vi "Activation Energies for 20201230.vi"() -> ()   [LabVIEW 2020]
uses:
  <vilib>/Analysis/NI_AALPro.lvlib
panel:
  in  "1/Temp 1D":dbl[](array[numeric])
  in  "ln|dG/dt| 1D":dbl[](array[numeric]) caption="ln|dG/dt|"
  out "E_a 1D HT":dbl
  in  "1/Temp lower temps 1D":dbl[](array[numeric])
  in  "ln|dG/dt| lower temps 1D":dbl[](array[numeric])
  out "E_a 1D":dbl
  out "Arrhenius 1D":T1(graph)
  out "Arrhenius":T1(graph)
  out "E_a 2":dbl
  in  "ln|dG/dt| lower temps":dbl[](array[numeric])
  in  "1/Temp lower temps":dbl[](array[numeric])
  out "E_a":dbl
  in  "ln|dG/dt|":dbl[](array[numeric])
  in  "1/Temp":dbl[](array[numeric])
  # "0.002817\t\n0.002778\t\n0.00274\t\n0.002703\t\n0.002667\t\n0.002632"
  # "0.003509\t\n0.003448\t\n0.00339\t\n0.003333\t\n0.003279\t\n0.003226\t\n0.003175\t\n0.003125\t\n0.003077\t\n0.00303"
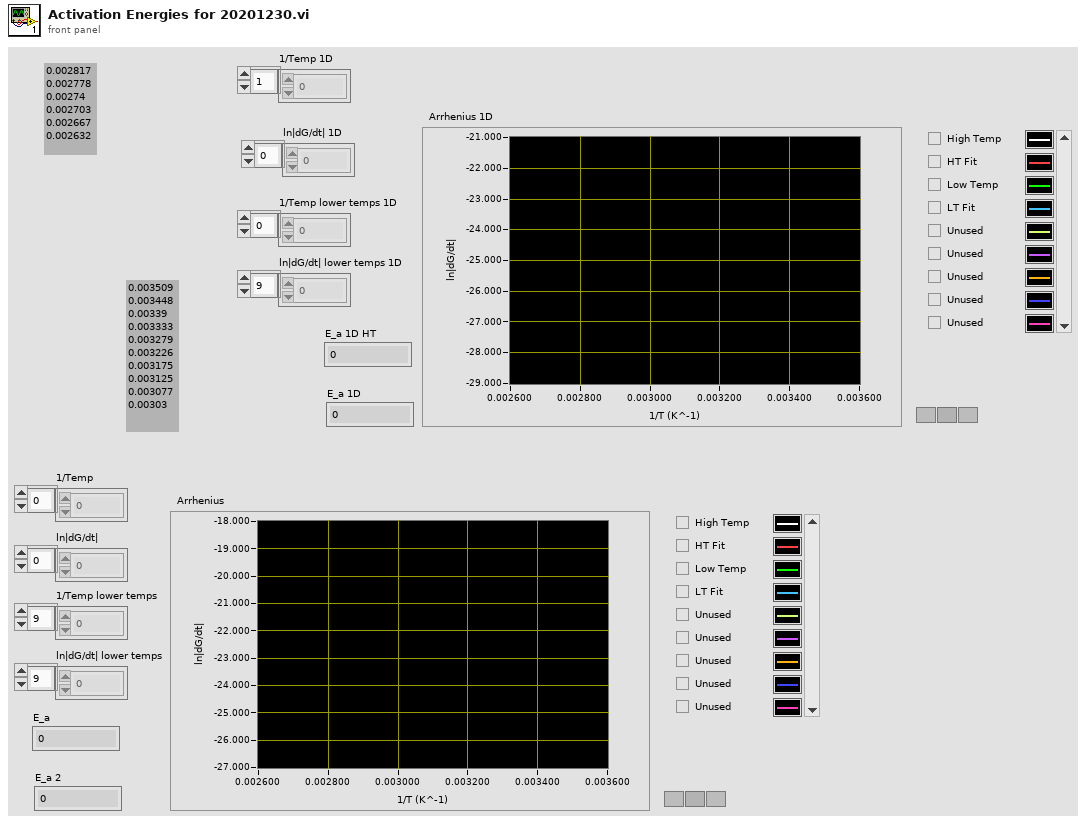
[diagram p1: front panel]
types:
  T1 = cluster{"Data":dbl[], "Best Exponential Fit":dbl[]}[]
  T2 = cluster{"1/Temp 1D":dbl[], "Best Linear Fit":dbl[]}
  T3 = cluster{"1/Temp lower temps 1D":dbl[], "ln|dG/dt| lower temps 1D":dbl[]}
  T4 = cluster{"1/Temp lower temps 1D":dbl[], "Best Linear Fit":dbl[]}
  T5 = cluster{"1/Temp lower temps 1D":dbl[], "Best Linear Fit":dbl[]}[]
  T6 = cluster{"1/Temp lower temps":dbl[], "ln|dG/dt| lower temps":dbl[]}
  T7 = cluster{"1/Temp lower temps":dbl[], "Best Linear Fit":dbl[]}
  T8 = cluster{"1/Temp lower temps":dbl[], "Best Linear Fit":dbl[]}[]
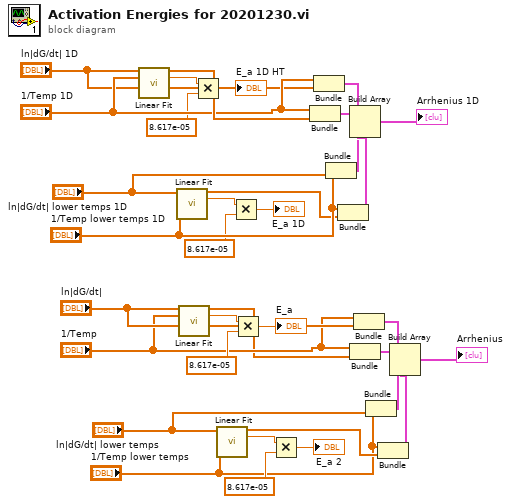
[diagram p0: block diagram]
diagram:
  n1 = call <vilib>:"Linear Fit.vi"("Y"="ln|dG/dt| 1D", "X"="1/Temp 1D") -> ("Best Linear Fit"=w15:dbl[], "slope"=w1:dbl)  [unwired: 9 in, 3 out]
  n2 = call <vilib>:"Linear Fit.vi"("Y"="ln|dG/dt| lower temps 1D", "X"="1/Temp lower temps 1D") -> ("Best Linear Fit"=w12:dbl[], "slope"=w6:dbl)  [unwired: 9 in, 3 out]
  n3 = call <vilib>:"Linear Fit.vi"("Y"="ln|dG/dt|", "X"="1/Temp") -> ("Best Linear Fit"=w20:dbl[], "slope"=w34:dbl)  [unwired: 9 in, 3 out]
  n4 = Multiply(x=w1, y=8.617e-05) -> (x*y=→"E_a 1D HT":dbl)
  n5 = call <vilib>:"Linear Fit.vi"("Y"="ln|dG/dt| lower temps", "X"="1/Temp lower temps") -> ("Best Linear Fit"=w23:dbl[], "slope"=w29:dbl)  [unwired: 9 in, 3 out]
  n6 = Multiply(x=w6, y=8.617e-05) -> (x*y=→"E_a 1D":dbl)
  n7 = Multiply(x=w34, y=8.617e-05) -> (x*y=→"E_a":dbl)
  n8 = Multiply(x=w29, y=8.617e-05) -> (x*y=→"E_a 2":dbl)
  n9 = Bundle("1/Temp 1D"="1/Temp 1D", "Best Linear Fit"=w15) -> (w16:T2)  [unwired: 1 in]
  n10 = Bundle("1/Temp 1D"="1/Temp 1D", "ln|dG/dt| 1D"="ln|dG/dt| 1D") -> (w9:cluster{"1/Temp 1D":dbl[], "ln|dG/dt| 1D":dbl[]})  [unwired: 1 in]
  n11 = Bundle("1/Temp lower temps 1D"="1/Temp lower temps 1D", "ln|dG/dt| lower temps 1D"="ln|dG/dt| lower temps 1D") -> (w11:T3)  [unwired: 1 in]
  n12 = Bundle("1/Temp lower temps 1D"="1/Temp lower temps 1D", "Best Linear Fit"=w12) -> (w17:T4)  [unwired: 1 in]
  n13 = Build Array(w9, w16, w11, w17) -> (→"Arrhenius 1D":T5)
  n14 = Bundle("1/Temp"="1/Temp", "Best Linear Fit"=w20) -> (w19:cluster{"1/Temp":dbl[], "Best Linear Fit":dbl[]})  [unwired: 1 in]
  n15 = Bundle("1/Temp"="1/Temp", "ln|dG/dt|"="ln|dG/dt|") -> (w26:cluster{"1/Temp":dbl[], "ln|dG/dt|":dbl[]})  [unwired: 1 in]
  n16 = Bundle("1/Temp lower temps"="1/Temp lower temps", "ln|dG/dt| lower temps"="ln|dG/dt| lower temps") -> (w24:T6)  [unwired: 1 in]
  n17 = Bundle("1/Temp lower temps"="1/Temp lower temps", "Best Linear Fit"=w23) -> (w18:T7)  [unwired: 1 in]
  n18 = Build Array(w26, w19, w24, w18) -> (→"Arrhenius":T8)
